vi "GenesysPS.i attribute.vi"(0 "VI Refnum":refnum<vi>, 2 "CLASS.i attribute":T1={"VISA name/ Heizinger"="", "GEN Addr"=1, "WithTempInt?"=FALSE, "TempLimit"=0.0, "TemperatureID"=0, "Temp queue"=refnum}, 3 "Action":T2(ring), 5 "error in (no error)":errorcluster) -> (14 "VI Refnum out":refnum<vi>, 16 "CLASS.i attribute out":T1={"VISA name/ Heizinger"="", "GEN Addr"=1, "WithTempInt?"=FALSE, "TempLimit"=0.0, "TemperatureID"=0, "Temp queue"=refnum}, 19 "error out":errorcluster)   [LabVIEW 2014, in "GenesysPS.lvlib"]
doc: "This is a so-called functional global variable. It manages the access to a global variable in a thread-safe way. \n\nHere the attribute data of all instances of THIS class are stored. This is done for performance reasons.\n\nLicense Agreement for this software:\n\nCopyright (C)\nGesellschaft für Schwerionenforschung, GSI\nPlanckstr. 1\n64291 Darmstadt\nGermany\n\nContact: D.Beck@gsi.de \n\nThis program is free software; you can redistribute it and/or modify it under the terms of the GNU General Public License as published by the Free Software Foundation; either version 2 of the license, or (at your option) any later version.\n\nThis program is distributed in the hope that it will be useful, but WITHOUT ANY WARRANTY; without even the implied warranty of MERCHANTABILITY or FITNESS FOR A PARTICULAR PURPOSE. See the GNU General License for more details (http://www.gnu.org).\n\nGesellschaft für Schwerionenforschung, GSI\nPlanckstr. 1, 64291 Darmstadt, Germany\nFor all questions and ideas contact: M.Richter@gsi.de, H.Brand@gsi.de or D.Beck@gsi.de.\nLast update: 17-JUN-2004"
uses:
  GenesysPS.lvlib
  GenesysPS.i attribute.ctl
  CS_Core/CSSystem/CoreDefs/CoreDefs.error_type.ctl
  CS_Core/CSSystem/CoreLib/CoreLib.lvlib
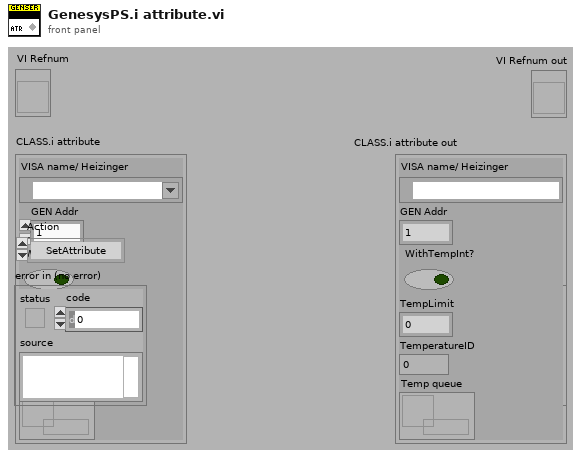
[diagram p1: front panel]
types:
  T1 = typedef "GenesysPS.lvlib/GenesysPS.i attribute.ctl" = cluster{"VISA name/ Heizinger":refnum<visa-resource-name>, "GEN Addr":i32, "WithTempInt?":bool, "TempLimit":dbl, "TemperatureID":i32, "Temp queue":refnum<queue>}
  T2 = enum16{"SetAttribute", "GetAttribute", "CreateAttribute", "DestroyAttribute", "DestroyAllAtributes"}
  T3 = typedef "CoreDefs.error_type.ctl" = enum16{"no error", "can't load process", "can't unload process", "process does not exist", "can't install process", "can't remove process", "unknown function", "time out", "can't execute function", "duplicate queue name", "super not found", "caller queue invalid", "can't ping process", "unknown error", "VISA Error", "VISA timeout", "GPIB timeout", "GPIB error", "communication error", "data type mismatch", "can't read data from OPC server", "can't write data to OPC server", "OET error", "function not implemented", "process already exists", "invalid Shared Variable name", "error writing Shared Variable", "error reading Shared Variable", "invalid client name", "corrupt database", "unknown class", "call not authorized", "parameter out of range", "OET timeout: can't get data to modify", "invalid queue name", "requested operation incompatible with current state", "event undefined", "event disabled", "state undefined", "caller is not a friend", "EventBuilder: bad eventID", "EventBuilder: no DAQ devices", "a thread must not stop itself", "UNUSED ELEMENT4", "DiscArchiver: eventData incomplete", "DiscArchiver: eventData does not belong to run", "DiscArchiver: can't open file", "DiscArchiver: can't write to file", "DiscArchiver: available disc space low", "can't acquire semaphore", "error reading data from database", "notifier object is not existing", "can't register process", "can't unregister process", "illegal event type", "object disabled", "object already exists", "can't change state", "Instrument not found", "no connection to remote node", "invalid reference", "N/A", "UNUSED ELEMENT 1", "element not found", "illegal TCP/IP connection detected", "object does not exist", "invalid access ID", "unknown CS system", "invalid privilige", "unsupported data type", "unsupported server type", "IO server already exists", "Shared Variable already exists"}
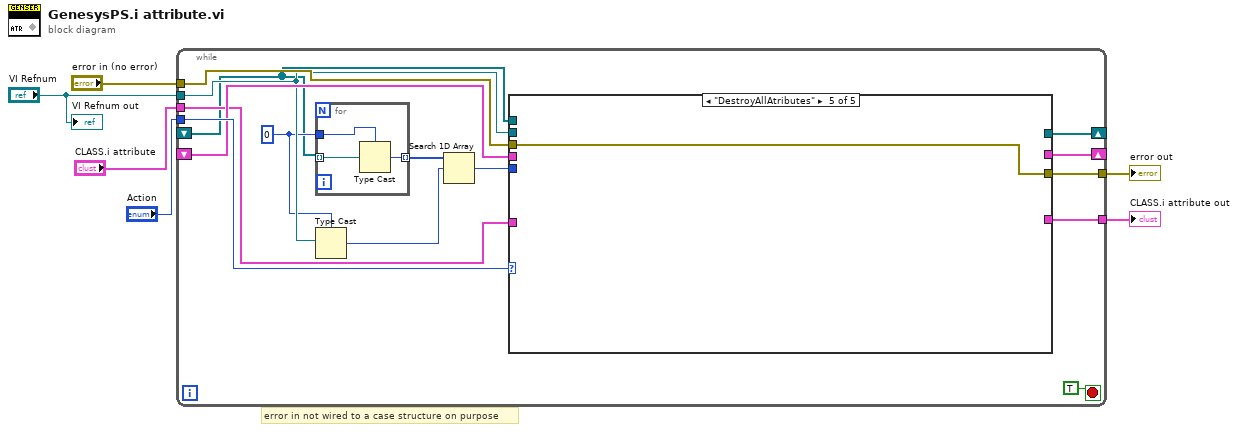
[diagram p0: block diagram]
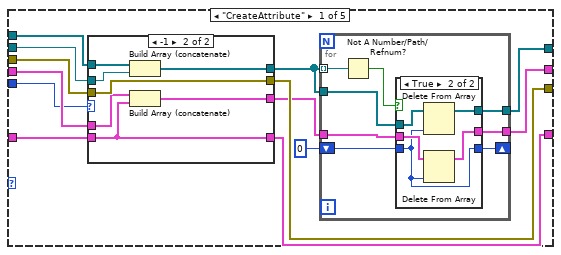
[diagram p2: hidden frame]
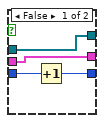
[diagram p3: hidden frame]
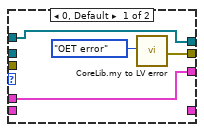
[diagram p4: hidden frame]
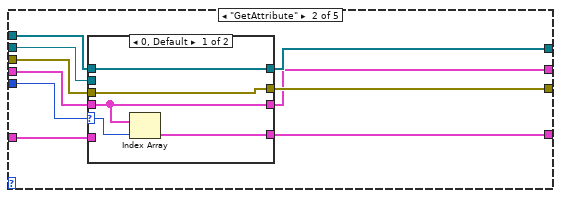
[diagram p5: hidden frame]
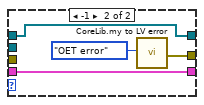
[diagram p6: hidden frame]
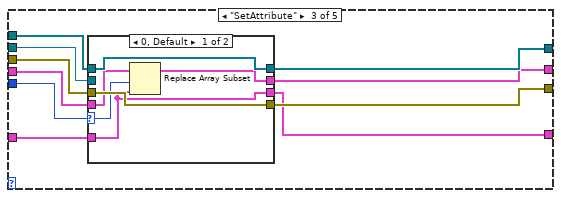
[diagram p7: hidden frame]
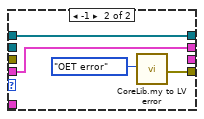
[diagram p8: hidden frame]
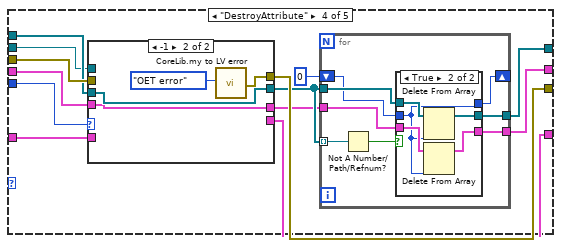
[diagram p9: hidden frame]
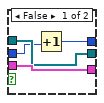
[diagram p10: hidden frame]
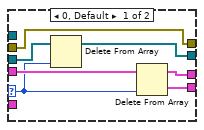
[diagram p11: hidden frame]
diagram:
  # "error in not wired to a case structure on purpose"
  n1 = while {
    shift-right: [w15] -> _
    shift-left: _ -> [w16]
    tunnel: "Action" -> [w20]
    shift-right: [w17] -> _
    shift-left: _ -> [w7]
    tunnel: "error in (no error)" -> [w19]
    tunnel: [w18] -> w4
    tunnel: "CLASS.i attribute" -> [w14]
    tunnel: [w12] -> w2
    tunnel: "VI Refnum" -> [w10]
    stop <- TRUE stop-if-true
    w9 = 0
    n2 = for {
      tunnel: w9 -> [w24]
      tunnel: [w23] -> w8 mode=indexing
      tunnel: w7 -> [w22] mode=indexing
      n3 = Type Cast(type=w24, x=w22) -> (*(type *) &x=w23:i32)
    }
    n4 = Type Cast(type=w9, x=w10) -> (*(type *) &x=w11:i32)
    n5 = Search 1D Array(1D array=w8, element=w11) -> (index of element=w13:i32)  [unwired: 1 in]
    n6 = case shown="\"DestroyAllAtributes\"" w20 {
      tunnel: w7 -> [w35 w73 w92 w115 _]
      tunnel: w10 -> [w34 w71 w90 w114 _]
      tunnel: w19 -> [w37 w75 w94 w117 w146]
      tunnel: [w36 w74 w93 w116 w146] -> w18
      tunnel: [w29 w72 w91 w109 _] -> w17
      tunnel: w16 -> [w33 w70 w89 w113 _]
      tunnel: [w28 w69 w88 w107 _] -> w15
      tunnel: w14 -> [w32 w68 w87 w112 _]
      tunnel: w13 -> [w31 w67 w86 w111 _]
      tunnel: [w25 w66 w85 w105 _] -> w12
      frame "CreateAttribute" {
        n7 = case shown="-1" w31 {
          tunnel: w37 -> [_ w65]
          tunnel: [w57 w65] -> w36
          tunnel: w35 -> [w56 w64]
          tunnel: [w56 w63] -> w27
          tunnel: w34 -> [_ w62]
          tunnel: w33 -> [w55 w61]
          tunnel: [w55 w60] -> w26
          tunnel: w32 -> [_ w59]
          tunnel: [_ w59] -> w25
          frame 0, Default {
            n8 = call "CoreLib.my to LV error.vi"("ErrorTypes"=CoreDefs.error_type."OET error") -> ("myErrorCluster"=w57:errorcluster)  [unwired: 17 in, 1 out]
          }
          frame -1 {
            n9 = Build Array (concatenate)(w64, w62) -> (w63:refnum<vi>[])
            n10 = Build Array (concatenate)(w61, w59) -> (w60:T1[])
          }
        }
        n11 = for {
          tunnel: w27 -> [w42]
          tunnel: [w41] -> w29
          tunnel: [w45] -> w28
          tunnel: w26 -> [w44]
          tunnel: w27 -> [w40] mode=indexing
          shift-right: [w39] -> _
          shift-left: 0 -> [w38]
          n12 = Not A Number/Path/Refnum?(number/path/refnum=w40) -> (NaN/Path/Refnum?=w43:bool)
          n13 = case shown="True" w43 {
            tunnel: [w49 w54] -> w45
            tunnel: w44 -> [w49 w53]
            tunnel: [w48 w51] -> w41
            tunnel: w42 -> [w48 w52]
            tunnel: w38 -> [w47 w50]
            tunnel: [w46 w50] -> w39
            frame False {
              n14 = Increment(x=w47) -> (x+1=w46:i32)
            }
            frame True {
              n15 = Delete From Array(array=w52, index=w50) -> (array with subset deleted=w51:refnum<vi>[])  [unwired: 1 in, 1 out]
              n16 = Delete From Array(array=w53, index=w50) -> (array with subset deleted=w54:T1[])  [unwired: 1 in, 1 out]
            }
          }
        }
      }
      frame "GetAttribute" {
        n17 = case shown="0, Default" w67 {
          selector: w67 -> [w78 _]
          tunnel: w75 -> [w80 _]
          tunnel: [w80 w83] -> w74
          tunnel: w73 -> [w79 w82]
          tunnel: [w79 w82] -> w72
          tunnel: w71 -> [_ _]
          tunnel: w70 -> [w77 w81]
          tunnel: [w77 w81] -> w69
          tunnel: w68 -> [_ _]
          tunnel: [w76 _] -> w66
          frame 0, Default {
            n18 = Index Array(array=w77, index=w78) -> (element=w76:T1)
          }
          frame -1 {
            n19 = call "CoreLib.my to LV error.vi"("ErrorTypes"=CoreDefs.error_type."OET error") -> ("myErrorCluster"=w83:errorcluster)  [unwired: 17 in, 1 out]
          }
        }
      }
      frame "SetAttribute" {
        n20 = case shown="0, Default" w86 {
          selector: w86 -> [w96 _]
          tunnel: w94 -> [w100 _]
          tunnel: [w100 w103] -> w93
          tunnel: w92 -> [w99 w102]
          tunnel: [w99 w102] -> w91
          tunnel: w90 -> [_ _]
          tunnel: w89 -> [w98 w101]
          tunnel: [w97 w101] -> w88
          tunnel: w87 -> [w95 _]
          tunnel: [w95 _] -> w85
          frame 0, Default {
            n21 = Replace Array Subset(array=w98, new element=w95, index=w96) -> (w97:T1[])
          }
          frame -1 {
            n22 = call "CoreLib.my to LV error.vi"("ErrorTypes"=CoreDefs.error_type."OET error") -> ("myErrorCluster"=w103:errorcluster)  [unwired: 17 in, 1 out]
          }
        }
      }
      frame "DestroyAttribute" {
        n23 = case shown="-1" w111 {
          selector: w111 -> [w137 _]
          tunnel: w117 -> [w141 _]
          tunnel: [w141 w144] -> w116
          tunnel: w115 -> [w140 w143]
          tunnel: [w139 w143] -> w108
          tunnel: w114 -> [_ _]
          tunnel: w113 -> [w138 w142]
          tunnel: [w136 w142] -> w106
          tunnel: w112 -> [_ _]
          tunnel: [w135 _] -> w105
          frame 0, Default {
            n24 = Delete From Array(array=w140, index=w137) -> (array with subset deleted=w139:refnum<vi>[])  [unwired: 1 in, 1 out]
            n25 = Delete From Array(array=w138, index=w137) -> (deleted portion=w135:T1, array with subset deleted=w136:T1[])  [unwired: 1 in]
          }
          frame -1 {
            n26 = call "CoreLib.my to LV error.vi"("ErrorTypes"=CoreDefs.error_type."OET error") -> ("myErrorCluster"=w144:errorcluster)  [unwired: 17 in, 1 out]
          }
        }
        n27 = for {
          tunnel: w108 -> [w122]
          tunnel: [w121] -> w109
          tunnel: [w125] -> w107
          tunnel: w106 -> [w124]
          tunnel: w108 -> [w120] mode=indexing
          shift-right: [w119] -> _
          shift-left: 0 -> [w118]
          n28 = Not A Number/Path/Refnum?(number/path/refnum=w120) -> (NaN/Path/Refnum?=w123:bool)
          n29 = case shown="True" w123 {
            tunnel: [w129 w134] -> w125
            tunnel: w124 -> [w129 w133]
            tunnel: [w128 w131] -> w121
            tunnel: w122 -> [w128 w132]
            tunnel: w118 -> [w127 w130]
            tunnel: [w126 w130] -> w119
            frame False {
              n30 = Increment(x=w127) -> (x+1=w126:i32)
            }
            frame True {
              n31 = Delete From Array(array=w132, index=w130) -> (array with subset deleted=w131:refnum<vi>[])  [unwired: 1 in, 1 out]
              n32 = Delete From Array(array=w133, index=w130) -> (array with subset deleted=w134:T1[])  [unwired: 1 in, 1 out]
            }
          }
        }
      }
      frame "DestroyAllAtributes" {
      }
    }
  }
  "error out" <- w4
  "CLASS.i attribute out" <- w2
  "VI Refnum out" <- "VI Refnum"
